vi "CreateDWarn.vi"(5 "Call Chain? (true)":bool=TRUE, 7 "DWarnInternal? (false)":bool, 8 "error in (no error)":errorcluster, 11 "DWarn Text":string) -> (0 "error out":errorcluster)   [LabVIEW 2020, in "NI_XNodeSupport.lvlib"]
uses:
  <vilib>/XNodeSupport/NI_XNodeSupport.lvlib
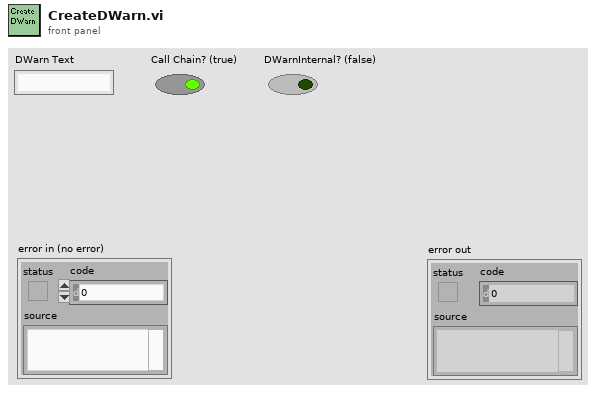
[diagram p1: front panel]
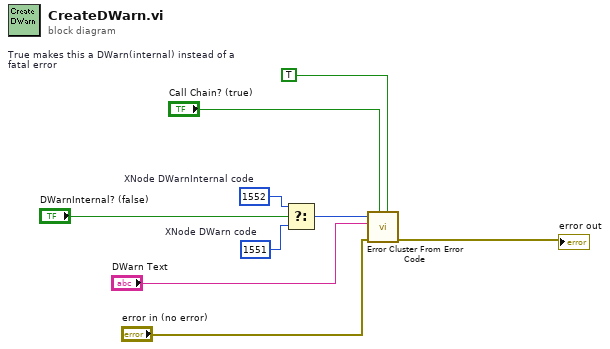
[diagram p0: block diagram]
diagram:
  w3 = 1552  # XNode DWarnInternal code
  w9 = TRUE  # True makes this a DWarn(internal) instead of a fatal error
  w4 = 1551  # XNode DWarn code
  n1 = Select(t=w3, s="DWarnInternal? (false)", f=w4) -> (s? t:f=w1:i32)
  n2 = call <vilib>:"Error Cluster From Error Code.vi"("is warning? (False)"=w9, "show call chain? (False)"="Call Chain? (true)", "error in (no error)"="error in (no error)", "error message (\"\")"="DWarn Text", "error code (0)"=w1) -> ("error out"=→"error out":errorcluster)  [unwired: 4 in]
